vi "LambdaMonitor.vi"   [LabVIEW 2016]
uses:
  Global/Global Variables/Data_Display_global.vi
  Instrument_Setup.vi
types:
  T1 = cluster{"Max 4.2K temp":dbl[unit], "Max 2.2K temp":dbl[unit], "Instrument address":cluster{"Com Port":i32, "ISOBUS Address":i32, "GPIB Address":i16, "Communication":enum16{"RS232", "ISOBUS", "GPIB", "Gateway"}}}
  T2 = cluster{"Com Port":i32, "ISOBUS Address":i32, "GPIB Address":i16, "Communication":enum16{"RS232", "ISOBUS", "GPIB", "Gateway"}}
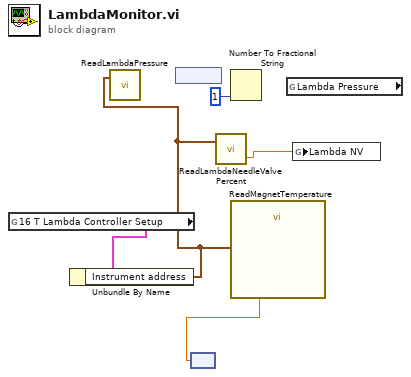
[diagram p0: block diagram]
diagram:
  n1 = global read "Instrument_Setup.vi" "16 T Lambda Controller Setup"() -> (w2:T1)
  n2 = Unbundle By Name(w2) -> ("Instrument address"=w1:T2)
  n3 = call "ReadLambdaPressure.vi"("Address"=w1) -> ()  [unwired: 1 in, 2 out]
  n4 = node() -> ()  [unwired: 1 in, 1 out]
  n5 = call "ReadLambdaNeedleValvePercent.vi"("Address"=w1) -> ("Actual Needle Valve  %"=w5:dbl)  [unwired: 1 in, 1 out]
  n6 = Number To Fractional String(precision (6)=1) -> ()  [unwired: 3 in, 1 out]
  n7 = call "ReadMagnetTemperature.vi"("Address"=w1) -> ("Magnet Temperature"=w7:dbl[unit])  [unwired: 1 in, 1 out]
  n8 = node(w7) -> (w3:dbl)
  n9 = global read "Data_Display_global.vi" "Lambda Pressure"() -> (w4:dbl)
  n10 = global write "Data_Display_global.vi" "Lambda NV"(w5) -> ()
